vi "NT Client_NoDS.vi"(4 "Update Time":i32=100, 9 "Client Name":string="Dashboard", 11 "TEAM":u32=4150) -> (0 "error out":errorcluster={"status"=FALSE, "code"=-1, "source"=""})   [LabVIEW 2019, in "Trajectory_Library.lvlib"]
doc: "Start a Network Tables client. Place this VI in the Dashboard or other client applications. Unlike the standard NT Client VI, this one does not need to run on the same computer as the driver station. This client determines the NT server (the robot's) IP address from the provided team number.\n\nThis VI does not run the NT client, it just starts it running. As such, it appears to return to the user after starting the NT client.\n\nInputs:\n - Team - U32 integer - Team number. This is used to determine the NT Server's IP address.\n - Client Name - string - Name of client sent to server. (I think). This can be anything. (Default: Dashboard)\n - Update Time - I32 integer - Time in milliseconds to update and get updates from the NT server. This can be specified as a smaller number for more time sensitive applications. (Default: 100)\n\nOutputs:\n - error out - error cluster - Reports if any errors occured."
uses:
  Trajectory_Library.lvlib
  <vilib>/Rock Robotics/Network Tables/NT Globals.vi
  FRC_NetworkTablesLV.dll
  ntcoreffi.dll
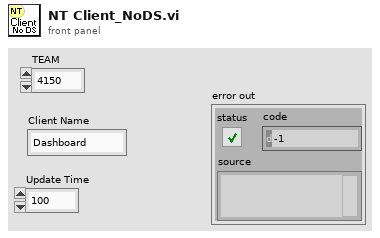
[diagram p1: front panel]
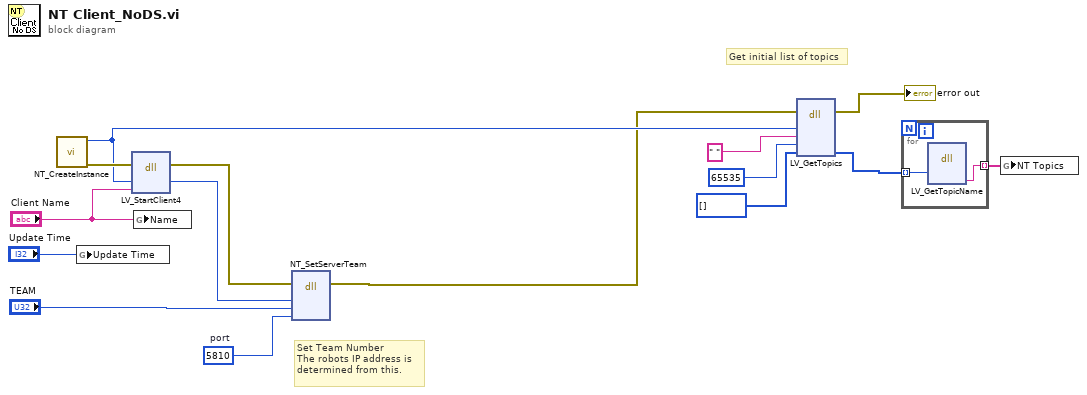
[diagram p0: block diagram]
diagram:
  w3 = u32 5810  # port
  # "Set Team Number\nThe robots IP address is \ndetermined from this."
  # "Get initial list of topics"
  n1 = call <vilib>:"NT_CreateInstance.vi"() -> ("error out"=w14:errorcluster, "InstanceHandle"=w12:u64)  [unwired: 10 in]
  n2 = global write "NT Globals.vi" "Update Time"("Update Time") -> ()
  n3 = dll-call lib="FRC_NetworkTablesLV.*" fn="LV_StartClient4"(error in=w14, "InstHandle"=w12, "identity"="Client Name") -> (error out=w6:errorcluster, "InstHandle"=w5:u64)  [unwired: 4 in, 1 out]
  n4 = global write "NT Globals.vi" "Name"("Client Name") -> ()
  n5 = dll-call lib="ntcoreffi.*" fn="NT_SetServerTeam"(error in=w6, "inst"=w5, "TEAM"="TEAM", "port"=w3) -> (error out=w1:errorcluster)  [unwired: 6 in, 1 out]
  n6 = dll-call lib="FRC_NetworkTablesLV.*" fn="LV_GetTopics"(error in=w1, "inst"=w12, "prefix"=" ", "typeMask"=u32 65535, "topicsArray"=u32[] []) -> (error out=→"error out":errorcluster, "topicsArray"=w9:u32[])  [unwired: 6 in, 1 out]
  n7 = for {
    tunnel: [w16] -> w10 mode=indexing
    tunnel: w9 -> [w17] mode=indexing
    n8 = dll-call lib="FRC_NetworkTablesLV.*" fn="LV_GetTopicName"("topic"=w17) -> ("name"=w16:string)  [unwired: 6 in, 2 out]
  }
  n9 = global write "NT Globals.vi" "NT Topics"(w10) -> ()
